vi "Update Default Value.vi"(8 "error in (no error)":errorcluster, 11 "List Data Type in":refnum<class "List Data Type.lvclass">) -> (0 "error out":errorcluster, 3 "List Data Type out":refnum<class "List Data Type.lvclass">)   [LabVIEW 2018, in "List Data Type.lvclass"]
uses:
  List Data Type.lvclass
  List Data Type.lvclass/List Data Type.ctl
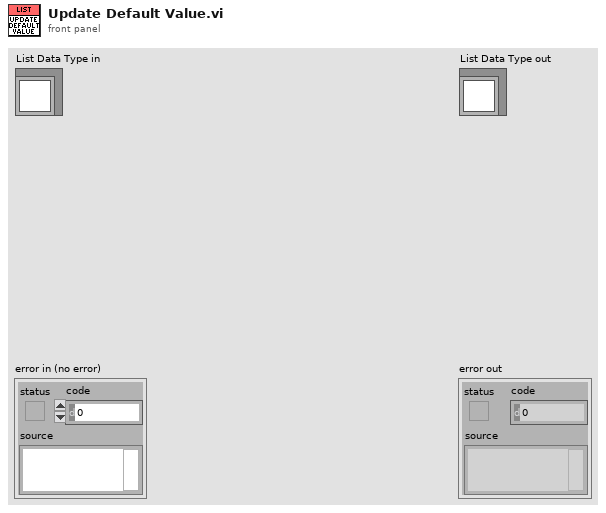
[diagram p1: front panel]
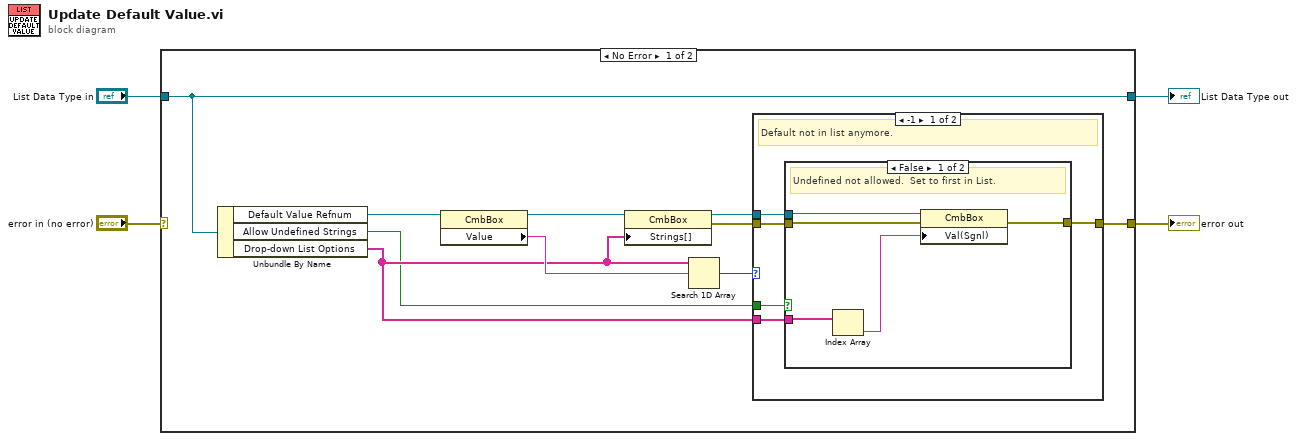
[diagram p0: block diagram]
diagram:
  n1 = case shown="No Error" "error in (no error)" {
    selector: "error in (no error)" -> [_ w28]
    tunnel: [w10 w28] -> w3
    tunnel: [w14 w27] -> w1
    tunnel: "List Data Type in" -> [w14 w27]
    frame No Error {
      n2 = Unbundle By Name(w14) -> ("Default Value Refnum"=w13:refnum<vi>, "Allow Undefined Strings"=w5:bool, "Drop-down List Options"=w8:string[])
      n3 = property class="CmbBox"(reference=w13) -> (reference out=w9:refnum<vi>, "Value"=w12:string)  [unwired: 1 in, 1 out]
      n4 = property class="CmbBox"(reference=w9, "Strings[]"=w8) -> (reference out=w7:refnum<vi>, error out=w6:errorcluster)  [unwired: 1 in]
      n5 = Search 1D Array(1D array=w8, element=w12) -> (index of element=w11:i32)  [unwired: 1 in]
      n6 = case shown="-1" w11 {
        tunnel: w7 -> [w18 _]
        tunnel: w6 -> [w17 w26]
        tunnel: [w15 w26] -> w10
        tunnel: w8 -> [w19 _]
        tunnel: w5 -> [w16 _]
        frame -1 {
          # "Default not in list anymore."
          n7 = case shown="False" w16 {
            tunnel: w19 -> [w22 _]
            tunnel: w18 -> [w24 _]
            tunnel: w17 -> [w23 w25]
            tunnel: [w20 w25] -> w15
            frame False {
              # "Undefined not allowed.  Set to first in List."
              n8 = Index Array(array=w22) -> (element=w21:string)  [unwired: 1 in]
              n9 = property class="CmbBox"(reference=w24, error in=w23, "Val(Sgnl)"=w21) -> (error out=w20:errorcluster)  [unwired: 1 out]
            }
            frame True {
              # "Undefined Strings are Allowed.  Do Nothing."
            }
          }
        }
        frame Default {
          # "Default is still in List.  Do Nothing."
        }
      }
    }
    frame Error {
    }
  }
  "error out" <- w3
  "List Data Type out" <- w1
